vi "Request Data JSON.vi"(8 "error in (no error)":errorcluster, 11 "GetSourceActive in":refnum<class "GetSourceActive.lvclass">) -> (0 "error out":errorcluster, 2 "Request Data JSON":string, 3 "GetSourceActive out":refnum<class "GetSourceActive.lvclass">)   [LabVIEW 2022 SP3, in "obs-websocket-lv.lvlib" / "GetSourceActive.lvclass"]
uses:
  GetSourceActive.lvclass
  GetSourceActive.lvclass/GetSourceActive.ctl
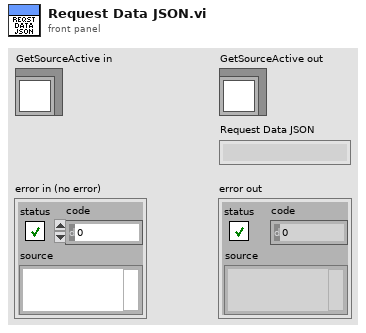
[diagram p1: front panel]
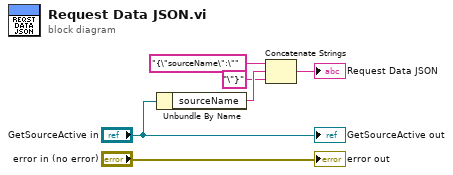
[diagram p0: block diagram]
diagram:
  n1 = Unbundle By Name("GetSourceActive in") -> ("sourceName"=w3:string)
  n2 = Concatenate Strings("{\"sourceName\":\"" ("string"), w3, "\"}" ("string")) -> (→"Request Data JSON":string)
  "error out" <- "error in (no error)"
  "GetSourceActive out" <- "GetSourceActive in"
